vi "3.2.vi"() -> ()   [LabVIEW 2019]
panel:
  out "y %":dbl
  out "Yn":dbl
  in  "x":dbl
  in  "N":dbl
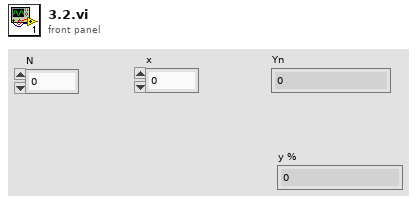
[diagram p1: front panel]
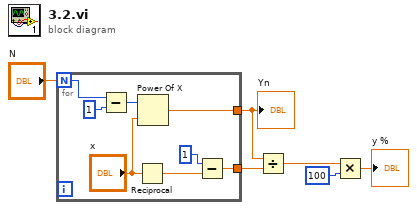
[diagram p0: block diagram]
diagram:
  n1 = for {
    N: "N" -> [w10]
    tunnel: [w13] -> w1
    tunnel: [w11] -> w2
    n2 = Subtract(x=w10, y=1) -> (x-y=w14:i32)
    n3 = Reciprocal(x="x") -> (1/x=w7:dbl)
    n4 = Power Of X(1:"x", 2:w14) -> (0:w13:dbl)
    n5 = Subtract(x=1, y=w7) -> (x-y=w11:dbl)
  }
  "Yn" <- w1
  n6 = Divide(x=w1, y=w2) -> (x/y=w5:dbl)
  n7 = Multiply(x=w5, y=100) -> (x*y=→"y %":dbl)
